vi "Measure Resistance Only_ERMod2.vi"(6 "Published_ID":string="_Free", 7 "Settings":T2 {"Sense" items=["Local"=1008, "Remote"=1009]}, 8 "error in (no error)":errorcluster, 9 "current level":dbl format="%_6p", 10 "Pins":string[](array[string]), 11 "Semiconductor Module Context":T3) -> (0 "error out":errorcluster, 3 "Semiconductor Module Context Out":T3)   [LabVIEW 2013]
uses:
  <vilib>/NI_TestStand_SemiconductorModule/NI_TestStand_Semiconductor_Module.lvlibp/PinMap/General/SemiconductorModuleContext.ctl
  <instrlib>/niDCPower/nidcpower.llb/niDCPower Sense.ctl
  <instrlib>/niDCPower/nidcpower.llb/niDCPower Wait For Event - Event.ctl
  <vilib>/NI_TestStand_SemiconductorModule/NI_TestStand_Semiconductor_Module.lvlibp/PinMap/DC Power/PinToNIDCPowerSessions.vi
  <vilib>/NI_TestStand_SemiconductorModule/NI_TestStand_Semiconductor_Module.lvlibp/PinMap/General/Publish/PublishDataDoubleFunctionalTest.vi
  <vilib>/NI_TestStand_SemiconductorModule/NI_TestStand_Semiconductor_Module.lvlibp
panel:
  out "R Array":dbl[](array[numeric])
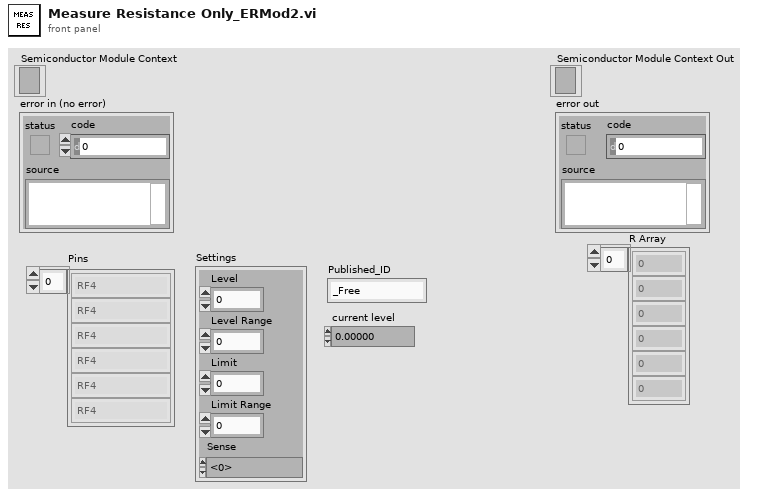
[diagram p1: front panel]
types:
  T1 = typedef "niDCPower Sense.ctl" = i32
  T2 = cluster{"Level":dbl, "Level Range":dbl, "Limit":dbl, "Limit Range":dbl, "Sense":T1}
  T3 = typedef "NI_TestStand_Semiconductor_Module.lvlibp/SemiconductorModuleContext.ctl" = refnum<k7>
  T4 = typedef "niDCPower Wait For Event - Event.ctl" = i32
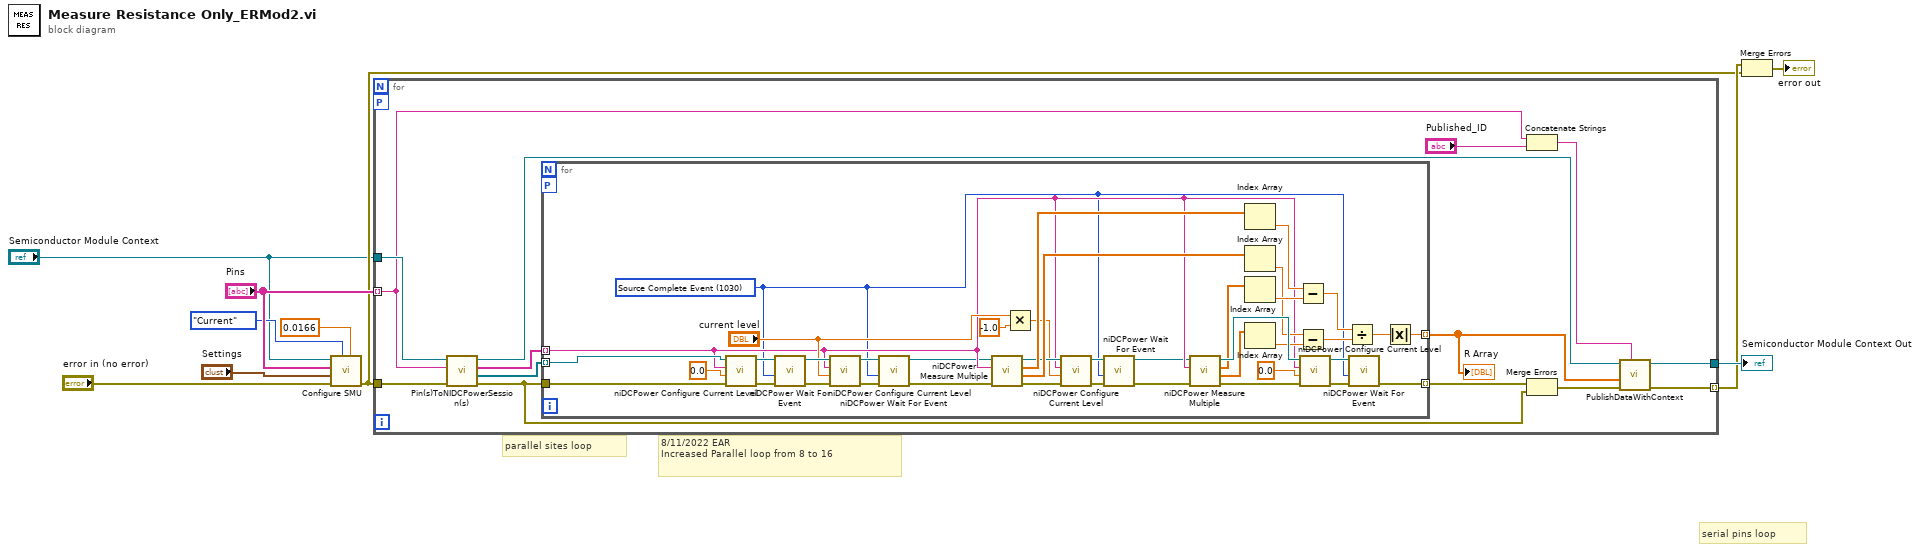
[diagram p0: block diagram]
diagram:
  # "8/11/2022 EAR\nIncreased Parallel loop from 8 to 16"
  # "parallel sites loop"
  # "serial pins loop"
  n1 = call "Configure SMU.vi"("aperture time"=0.0166, "Source Mode"=enum16{"Voltage", "Current"}."Current", "error in (no error)"="error in (no error)", "Settings"="Settings", "Pins"="Pins", "Semiconductor Module Context"="Semiconductor Module Context") -> ("error out"=w5:errorcluster)  [unwired: 5 in]
  n2 = for {
    tunnel: "Semiconductor Module Context" -> [w23]
    tunnel: [w17] -> w10
    tunnel: "Pins" -> [w14] mode=indexing
    tunnel: w5 -> [w24]
    tunnel: [w15] -> w8 mode=indexing
    workers-P: _ -> [_]
    n3 = call-poly <vilib>:"Pin(s)ToNIDCPowerSession(s).vi"("error in (no error)"=w24, "Pin"=w14, "Semiconductor Module Context"=w23) -> ("error out"=w19:errorcluster, "Instrument Sessions"=w21:refnum<k15>[], "Channel Lists"=w22:string[], "Semiconductor Module Context Out"=w18:T3)  [unwired: 4 in, 1 out]
    n4 = for {
      tunnel: w22 -> [w30] mode=indexing
      tunnel: w21 -> [w48] mode=indexing
      workers-P: _ -> [_]
      tunnel: w19 -> [w53]
      tunnel: [w63] -> w20 mode=indexing
      tunnel: [w55] -> w11 mode=indexing
      w29 = T4 1030 items=["Source Complete Event"=1030, "Measure Complete Event"=1031, "Sequence Iteration Complete Event"=1032, "Sequence Engine Done Event"=1033, "Pulse Complete Event"=1051, "Ready For Pulse Trigger Event"=1052] ("event")
      n5 = call <instrlib>:"niDCPower Configure Current Level.vi"("error in (no error)"=w53, "current level"=0.0, "channel name"=w30, "instrument handle"=w48) -> ("error out"=w52:errorcluster, "instrument handle out"=w50:refnum<k15>)  [unwired: 6 in]
      n6 = call <instrlib>:"niDCPower Wait For Event.vi"("error in (no error)"=w52, "event"=w29, "instrument handle"=w50) -> ("error out"=w51:errorcluster, "instrument handle out"=w49:refnum<k15>)  [unwired: 7 in]
      n7 = call <instrlib>:"niDCPower Configure Current Level.vi"("error in (no error)"=w51, "current level"="current level", "channel name"=w30, "instrument handle"=w49) -> ("error out"=w60:errorcluster, "instrument handle out"=w59:refnum<k15>)  [unwired: 6 in]
      n8 = call <instrlib>:"niDCPower Wait For Event.vi"("error in (no error)"=w60, "event"=w29, "instrument handle"=w59) -> ("error out"=w28:errorcluster, "instrument handle out"=w27:refnum<k15>)  [unwired: 7 in]
      n9 = call <instrlib>:"niDCPower Measure Multiple.vi"("error in (no error)"=w28, "channel name"=w30, "instrument handle"=w27) -> ("error out"=w43:errorcluster, "current measurements"=w56:dbl[], "voltage measurements"=w57:dbl[], "instrument handle out"=w41:refnum<k15>)  [unwired: 5 in]
      n10 = Multiply(x="current level", y=-1.0) -> (x*y=w31:dbl)
      n11 = call <instrlib>:"niDCPower Configure Current Level.vi"("error in (no error)"=w43, "current level"=w31, "channel name"=w30, "instrument handle"=w41) -> ("error out"=w45:errorcluster, "instrument handle out"=w44:refnum<k15>)  [unwired: 6 in]
      n12 = call <instrlib>:"niDCPower Wait For Event.vi"("error in (no error)"=w45, "event"=w29, "instrument handle"=w44) -> ("error out"=w26:errorcluster, "instrument handle out"=w25:refnum<k15>)  [unwired: 7 in]
      n13 = call <instrlib>:"niDCPower Measure Multiple.vi"("error in (no error)"=w26, "channel name"=w30, "instrument handle"=w25) -> ("error out"=w42:errorcluster, "current measurements"=w38:dbl[], "voltage measurements"=w39:dbl[], "instrument handle out"=w40:refnum<k15>)  [unwired: 5 in]
      n14 = Index Array(array=w57) -> (element=w37:dbl)  [unwired: 1 in]
      n15 = Index Array(array=w56) -> (element=w35:dbl)  [unwired: 1 in]
      n16 = Index Array(array=w39) -> (element=w36:dbl)  [unwired: 1 in]
      n17 = Index Array(array=w38) -> (element=w34:dbl)  [unwired: 1 in]
      n18 = Subtract(x=w37, y=w36) -> (x-y=w33:dbl)
      n19 = Subtract(x=w35, y=w34) -> (x-y=w32:dbl)
      n20 = call <instrlib>:"niDCPower Configure Current Level.vi"("error in (no error)"=w42, "current level"=0.0, "channel name"=w30, "instrument handle"=w40) -> ("error out"=w64:errorcluster, "instrument handle out"=w62:refnum<k15>)  [unwired: 6 in]
      n21 = Divide(x=w33, y=w32) -> (x/y=w58:dbl)
      n22 = call <instrlib>:"niDCPower Wait For Event.vi"("error in (no error)"=w64, "event"=w29, "instrument handle"=w62) -> ("error out"=w63:errorcluster)  [unwired: 7 in, 1 out]
      n23 = Absolute Value(x=w58) -> (abs(x)=w55:dbl)
    }
    "R Array" <- w11
    n24 = Concatenate Strings(w14, "Published_ID") -> (w12:string)
    n25 = Merge Errors(w20, w19) -> (w16:errorcluster)
    n26 = call-poly <vilib>:"PublishDataWithContext.vi"("Published Data Id"=w12, "error in (no error)"=w16, "Data In"=w11, "Semiconductor Module Context"=w18) -> ("error out"=w15:errorcluster, "Semiconductor Module Context Out"=w17:T3)  [unwired: 6 in]
  }
  "Semiconductor Module Context Out" <- w10
  n27 = Merge Errors(w8, w5) -> (→"error out":errorcluster)
